vi "Configure Temperature (FRTD).vi"(0 "VISA resource name":refnum<visa-resource-name>, 5 "FRTD Type (0: Type 85)":u16(ring) items=["Type 85", "Type 91"], 7 "FRTD Reference (10)":dbl=10.0, 9 "Units (0: Celsius)":u16(ring) items=["Celsius", "Fahrenheit", "Kelvin"], 11 "error in (no error)":errorcluster) -> (4 "VISA resource name out":refnum<visa-resource-name>, 15 "error out":errorcluster)   [LabVIEW 2021, in "Agilent 34420.lvlib"]
doc: "Configures four wire RTD settings for temperature measurements."
uses:
  <instrlib>/Agilent 34420/Agilent 34420.lvlib
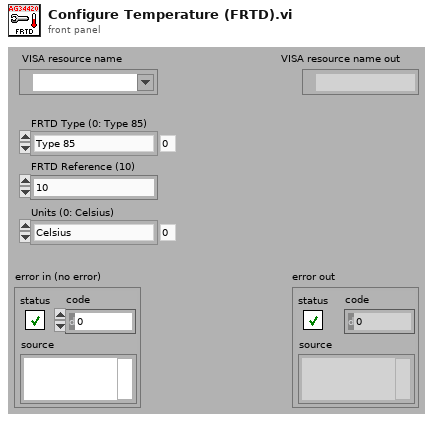
[diagram p1: front panel]
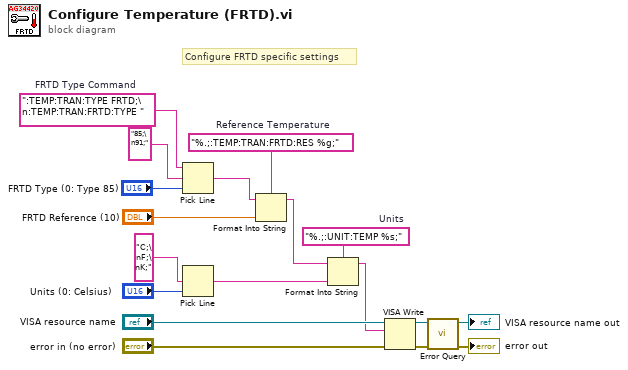
[diagram p0: block diagram]
diagram:
  w2 = "%.;:UNIT:TEMP %s;"  # Units
  w7 = "%.;:TEMP:TRAN:FRTD:RES %g;"  # Reference Temperature
  w11 = ":TEMP:TRAN:TYPE FRTD;\n:TEMP:TRAN:FRTD:TYPE "  # FRTD Type Command
  # "Configure FRTD specific settings"
  n1 = Pick Line(string ("")=w11, multi-line string="85;\n91;", line index="FRTD Type (0: Type 85)") -> (output string=w8:string)
  n2 = Pick Line(multi-line string="C;\nF;\nK;", line index="Units (0: Celsius)") -> (output string=w4:string)  [unwired: 1 in]
  n3 = Format Into String(format string=w7, initial string=w8, "FRTD Reference (10)") -> (resulting string=w3:string)  [unwired: 1 in, 1 out]
  n4 = Format Into String(format string=w2, initial string=w3, w4) -> (resulting string=w1:string)  [unwired: 1 in, 1 out]
  n5 = VISA Write(VISA resource name="VISA resource name", write buffer=w1, error in (no error)="error in (no error)") -> (VISA resource name out=w14:refnum<visa-resource-name>, error out=w13:errorcluster)  [unwired: 1 out]
  n6 = call <instrlib>:"Error Query.vi"("error in (no error)"=w13, "VISA resource name"=w14) -> ("error out"=→"error out":errorcluster, "VISA resource name out"=→"VISA resource name out":refnum<visa-resource-name>)  [unwired: 6 in, 2 out]
